vi "ReadLatest.vi"(0 "object in":refnum<class "CoriFlowBFS1Plus.lvclass">, 5 "error in (no error)":errorcluster) -> (14 "object out":refnum<class "CoriFlowBFS1Plus.lvclass">, 16 "Latest Data":T1, 19 "error out":errorcluster)   [LabVIEW 2021, in "CoriFlowBFS1Plus.lvclass"]
uses:
  CoriFlowBFS1Plus.lvclass
  CoriFlowBFS1Plus.lvclass/CoriFlowBFS1Plus.ctl
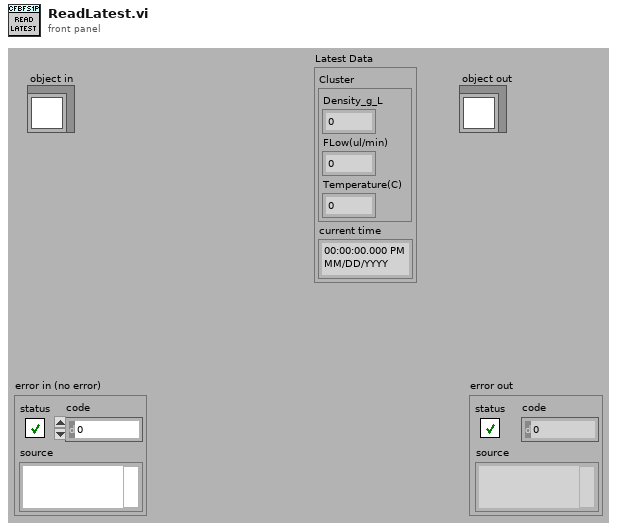
[diagram p1: front panel]
types:
  T1 = cluster{"Cluster":cluster{"Density_g_L":sgl, "FLow(ul/min)":sgl, "Temperature(C)":sgl}, "current time":timestamp}
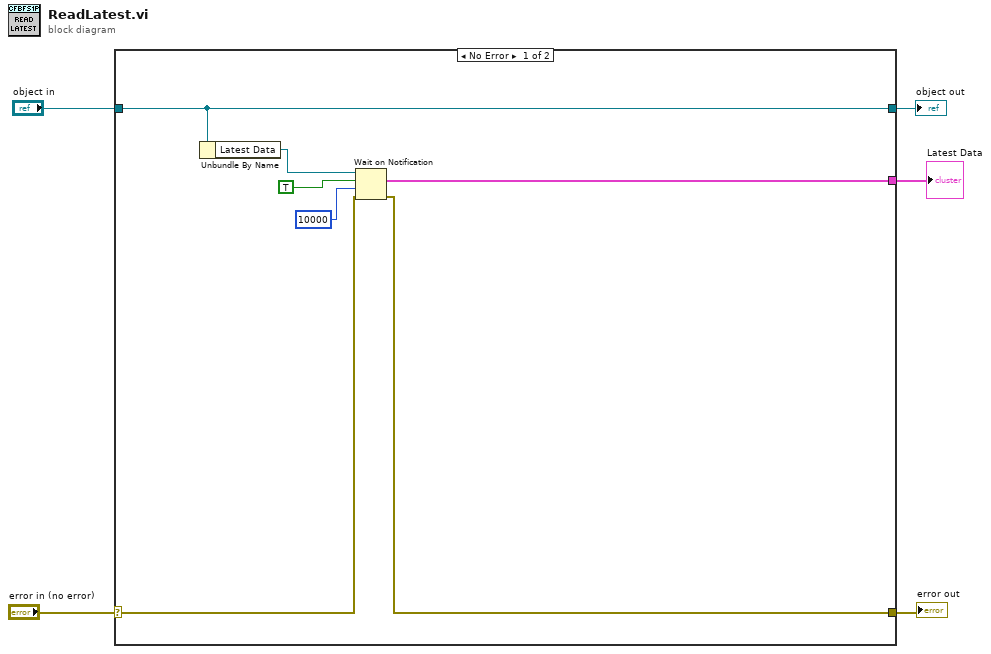
[diagram p0: block diagram]
diagram:
  n1 = case shown="No Error" "error in (no error)" {
    selector: "error in (no error)" -> [w10 w14]
    tunnel: [w9 w14] -> w4
    tunnel: [w12 w13] -> w2
    tunnel: "object in" -> [w12 w13]
    tunnel: [w7 _] -> w1
    frame No Error {
      n2 = Unbundle By Name(w12) -> ("Latest Data"=w11:refnum<notifier>)
      n3 = Wait on Notification(notifier=w11, ignore previous (F)=TRUE, timeout in ms (-1)=10000, error in (no error)=w10) -> (notification=w7:T1, error out=w9:errorcluster)  [unwired: 2 out]
    }
    frame Error {
    }
  }
  "error out" <- w4
  "object out" <- w2
  "Latest Data" <- w1
